vi "Read Valid Messages.vi"(8 "error in (no error)":errorcluster, 11 "controller in":refnum<class "LC Parser.lvclass">) -> (0 "error out":errorcluster, 2 "Valid Messages":string[](array[string]), 3 "controller out":refnum<class "LC Parser.lvclass">)   [LabVIEW 2020, in "LC Parser.lvclass"]
uses:
  LC Parser.lvclass
  Controller/Generic Plugin.lvclass
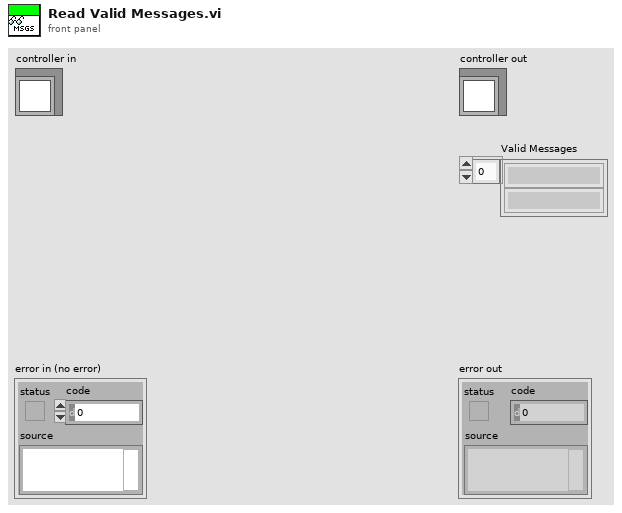
[diagram p1: front panel]
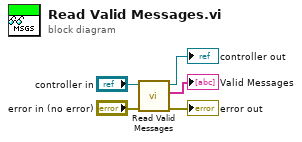
[diagram p0: block diagram]
diagram:
  n1 = call-parent "Read Valid Messages.vi"("error in (no error)"="error in (no error)", "controller in"="controller in") -> ("error out"=→"error out":errorcluster, "Valid Messages"=→"Valid Messages":string[], "controller out"=→"controller out":refnum<class "LC Parser.lvclass">)  [unwired: 7 in]
